vi "CPP-BLNormaliseToZref.vi"() -> (0 "New Values In":string[][](array[string]), 1 "New Chs In":string[](array[string]))   [LabVIEW 2018]
uses:
  Results_plotter_Global.vi
  Data plotting/subVIs/Plot_Values_Global.vi
panel:
  in  "Zref":dbl=1000.0
  # "This VI receives \"classic\" transposed plots of U/Uref vs Z, and linearly interpolates to find a velocity at a given height.\nFor use when re-normalising profiles about a height other than their original reference.\nTry a test run first and set Zref as required before processing a batch of profiles!"
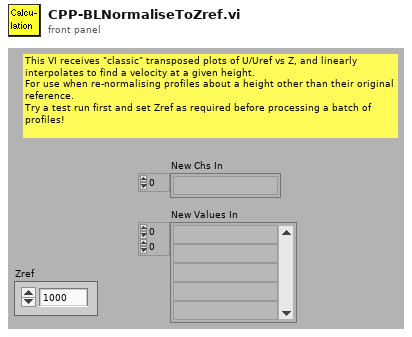
[diagram p1: front panel]
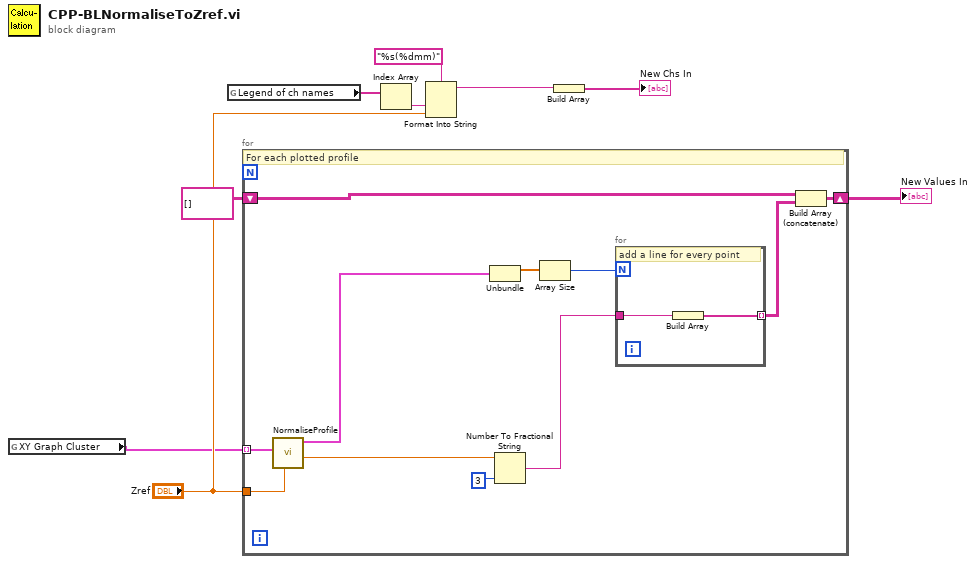
[diagram p0: block diagram]
diagram:
  n1 = global read "Plot_Values_Global.vi" "XY Graph Cluster"() -> (w1:cluster{dbl[], dbl[]}[])
  n2 = global read "Results_plotter_Global.vi" "Legend of ch names"() -> (w4:string[])
  n3 = for {
    tunnel: "Zref" -> [w12]
    tunnel: w1 -> [w13] mode=indexing
    shift-right: [w18] -> w7
    shift-left: string[][] [] -> [w17]
    # "For each plotted profile"
    n4 = call "NormaliseProfile.vi"("Zref"=w12, "UzClusterIn"=w13) -> ("U(Zref)"=w11:dbl, "UzClusterOutput"=w10:cluster{dbl[], dbl[]})  [unwired: 8 in]
    n5 = Unbundle(w10) -> (w15:dbl[])  [unwired: 1 out]
    n6 = Number To Fractional String(number=w11, precision (6)=i16 3) -> (F-format string=w19:string)  [unwired: 2 in]
    n7 = Array Size(array=w15) -> (size(s)=w16:i32)
    n8 = for {
      N: w16 -> [_]
      tunnel: w19 -> [w22]
      tunnel: [w21] -> w14 mode=indexing
      # "add a line for every point"
      n9 = Build Array(w22) -> (w21:string[])
    }
    n10 = Build Array (concatenate)(w17, w14) -> (w18:string[][])
  }
  "New Values In" <- w7
  n11 = Index Array(array=w4) -> (element=w2:string)  [unwired: 1 in]
  n12 = Format Into String(format string="%s(%dmm)", w2, "Zref") -> (resulting string=w6:string)  [unwired: 2 in, 1 out]
  n13 = Build Array(w6) -> (→"New Chs In":string[])
